vi "Red ball detection subVI.vi"(2 "error in":errorcluster, 3 "Image In":T1) -> (0 "error out":errorcluster, 1 "Image overlay":T1(plugin-control))   [LabVIEW 2018]
uses:
  <vilib>/vision/Image Controls.llb/IMAQ Image.ctl
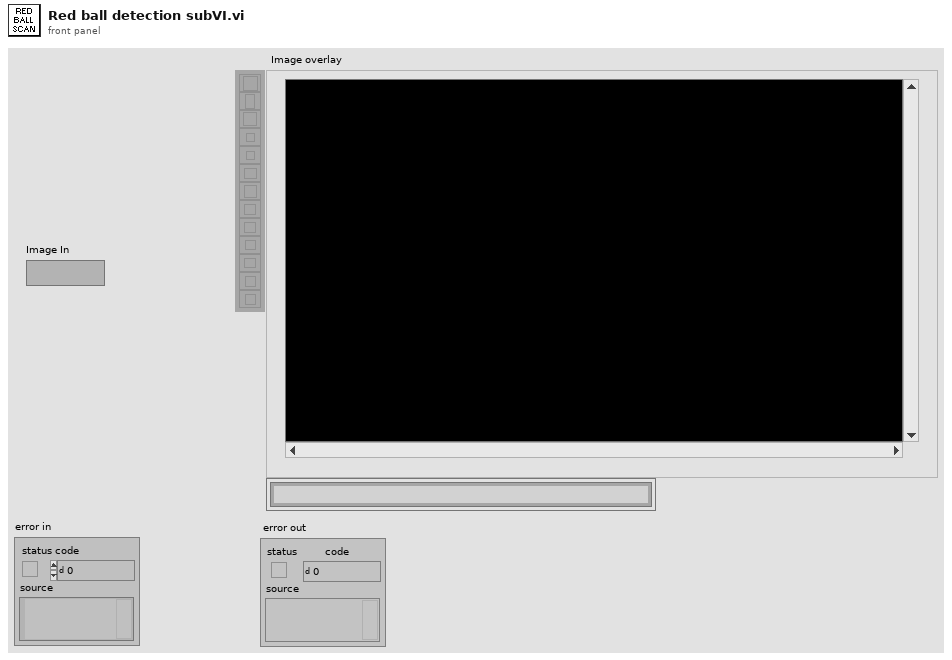
[diagram p1: front panel]
types:
  T1 = typedef "IMAQ Image.ctl" = refnum<image>
  T2 = cluster{"Desired Font (Application)":enum16{"User-specified Font", "Application Font", "System Font", "Dialog Font"}, "[User-specified Font]":cluster{"Font Name":string, "Size":i16, "Strikeout?":bool, "Italic?":bool, "Underline?":bool, "Outline?":bool, "Shadow?":bool, "Bold?":bool, "Rotation Angle":dbl}, "Horizontal Alignment":i16, "Vertical Alignment":i16}
  T3 = cluster{"Position":cluster{"x":sgl, "y":sgl}, "Angle":sgl, "Scale":sgl, "Score":sgl, "Bounding Box":cluster{"x":sgl, "y":sgl}[]}[]
  T4 = cluster{"Matches (Detect red)[0]":cluster{"Position":cluster{"x":sgl, "y":sgl}, "Angle":sgl, "Scale":sgl, "Score":sgl, "Bounding Box":cluster{"x":sgl, "y":sgl}[]}, "Matches (Detect red)[1]":cluster{"Position":cluster{"x":sgl, "y":sgl}, "Angle":sgl, "Scale":sgl, "Score":sgl, "Bounding Box":cluster{"x":sgl, "y":sgl}[]}, "Matches (Detect red)[2]":cluster{"Position":cluster{"x":sgl, "y":sgl}, "Angle":sgl, "Scale":sgl, "Score":sgl, "Bounding Box":cluster{"x":sgl, "y":sgl}[]}, "Matches (Detect red)[3]":cluster{"Position":cluster{"x":sgl, "y":sgl}, "Angle":sgl, "Scale":sgl, "Score":sgl, "Bounding Box":cluster{"x":sgl, "y":sgl}[]}, "Matches (Detect red)[4]":cluster{"Position":cluster{"x":sgl, "y":sgl}, "Angle":sgl, "Scale":sgl, "Score":sgl, "Bounding Box":cluster{"x":sgl, "y":sgl}[]}, "Matches (Detect red)[5]":cluster{"Position":cluster{"x":sgl, "y":sgl}, "Angle":sgl, "Scale":sgl, "Score":sgl, "Bounding Box":cluster{"x":sgl, "y":sgl}[]}, "Matches (Detect red)[6]":cluster{"Position":cluster{"x":sgl, "y":sgl}, "Angle":sgl, "Scale":sgl, "Score":sgl, "Bounding Box":cluster{"x":sgl, "y":sgl}[]}, "Matches (Detect red)[7]":cluster{"Position":cluster{"x":sgl, "y":sgl}, "Angle":sgl, "Scale":sgl, "Score":sgl, "Bounding Box":cluster{"x":sgl, "y":sgl}[]}, "Matches (Detect red)[8]":cluster{"Position":cluster{"x":sgl, "y":sgl}, "Angle":sgl, "Scale":sgl, "Score":sgl, "Bounding Box":cluster{"x":sgl, "y":sgl}[]}}
  T5 = cluster{"Bounding Box[0]":cluster{"x":sgl, "y":sgl}, "Bounding Box[1]":cluster{"x":sgl, "y":sgl}, "Bounding Box[2]":cluster{"x":sgl, "y":sgl}, "Bounding Box[3]":cluster{"x":sgl, "y":sgl}, "Bounding Box[4]":cluster{"x":sgl, "y":sgl}, "Bounding Box[5]":cluster{"x":sgl, "y":sgl}, "Bounding Box[6]":cluster{"x":sgl, "y":sgl}, "Bounding Box[7]":cluster{"x":sgl, "y":sgl}, "Bounding Box[8]":cluster{"x":sgl, "y":sgl}}
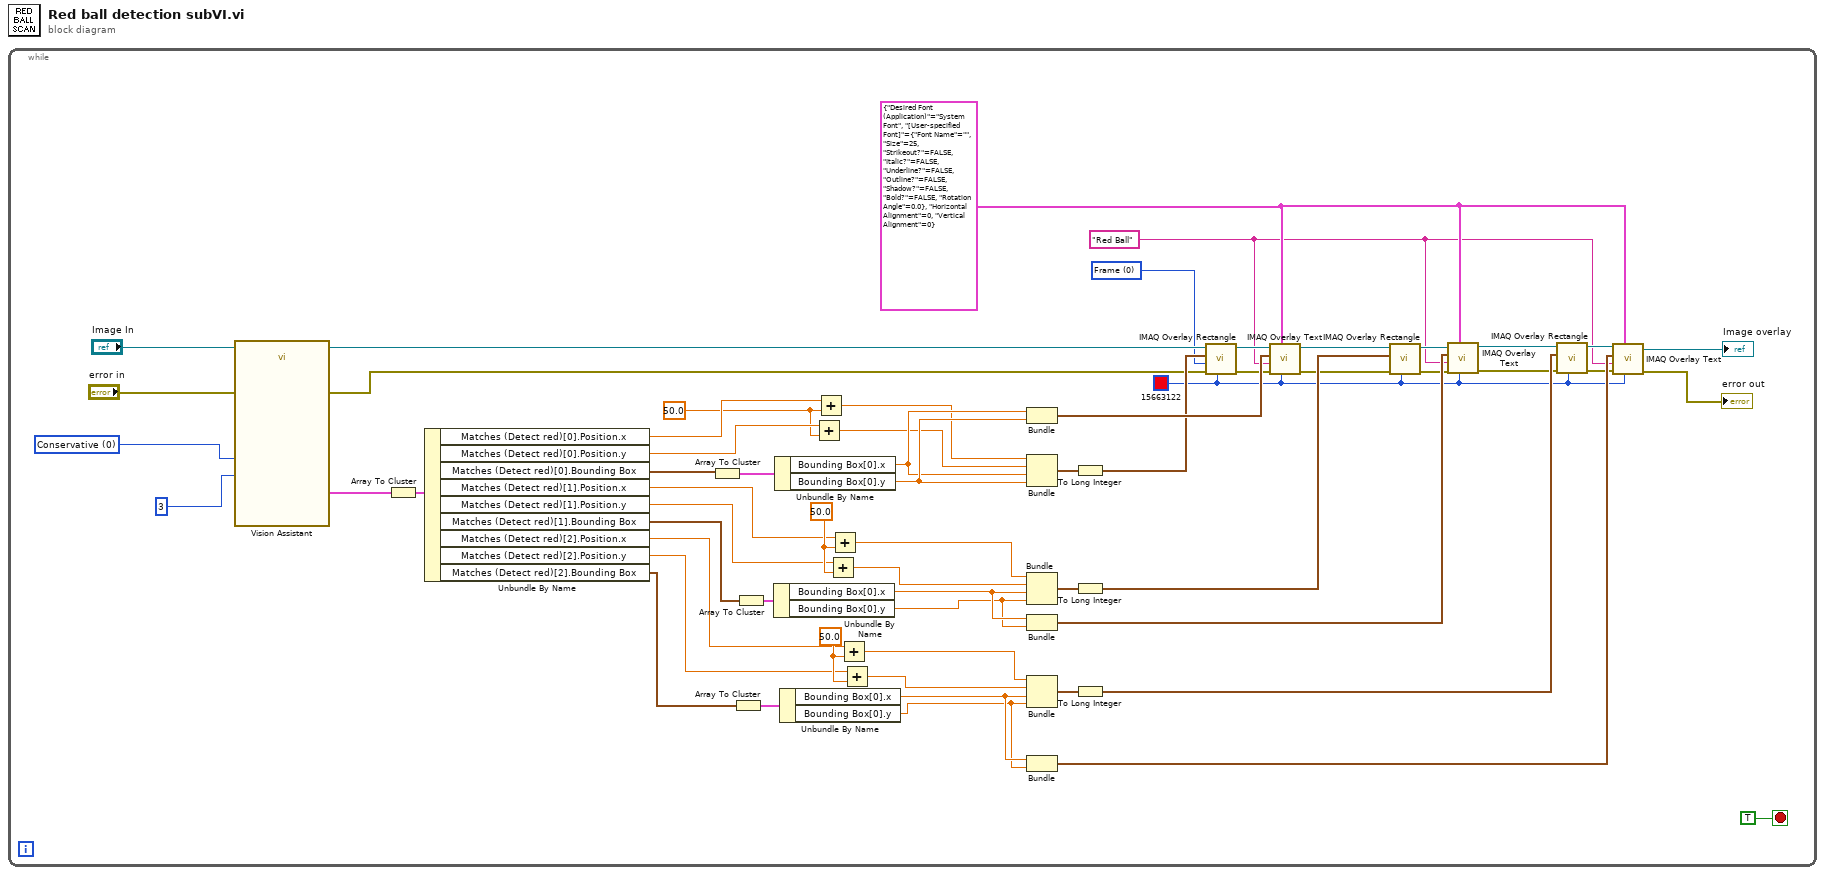
[diagram p0: block diagram]
diagram:
  n1 = while {
    stop <- TRUE stop-if-true
    w45 = u32 0 items=["Conservative", "Balance", "Aggressive", "Very Aggressive"] ("Search Strategy (Detect red)")
    w25 = sgl 50.0 ("y")
    w40 = sgl 50.0 ("y")
    w41 = sgl 50.0 ("y")
    w1 = u32 15663122 ("Text Color (black)")
    w13 = T2 {"Desired Font (Application)"=enum."System Font", "[User-specified Font]"={"Font Name"="", "Size"=25, "Strikeout?"=FALSE, "Italic?"=FALSE, "Underline?"=FALSE, "Outline?"=FALSE, "Shadow?"=FALSE, "Bold?"=FALSE, "Rotation Angle"=0.0}, "Horizontal Alignment"=0, "Vertical Alignment"=0} ("Font, Size & Style")
    w12 = "Red Ball" ("String")
    w33 = u32 0 items=["Frame", "Fill", "Highlight"] ("Drawing Mode (Frame)")
    n2 = call "Vision Assistant"("Image In"="Image In", "Search Strategy (Detect red)"=w45, "Number of Matches Requested (Detect red)"=3, "error in"="error in") -> ("Image Out"=w58:T1, "Matches (Detect red)"=w60:T3, "error out"=w2:errorcluster)  [unwired: 20 in, 1 out]
    n3 = Array To Cluster(array=w60) -> (cluster=w59:T4)
    n4 = Unbundle By Name(w59) -> ("Matches (Detect red)[0].Position.x"=w49:sgl, "Matches (Detect red)[0].Position.y"=w47:sgl, "Matches (Detect red)[0].Bounding Box"=w57:cluster{"x":sgl, "y":sgl}[], "Matches (Detect red)[1].Position.x"=w39:sgl, "Matches (Detect red)[1].Position.y"=w38:sgl, "Matches (Detect red)[1].Bounding Box"=w43:cluster{"x":sgl, "y":sgl}[], "Matches (Detect red)[2].Position.x"=w24:sgl, "Matches (Detect red)[2].Position.y"=w23:sgl, "Matches (Detect red)[2].Bounding Box"=w26:cluster{"x":sgl, "y":sgl}[])
    n5 = Array To Cluster(array=w57) -> (cluster=w56:T5)
    n6 = Array To Cluster(array=w26) -> (cluster=w27:T5)
    n7 = Array To Cluster(array=w43) -> (cluster=w42:T5)
    n8 = Unbundle By Name(w42) -> ("Bounding Box[0].x"=w30:sgl, "Bounding Box[0].y"=w29:sgl)
    n9 = Unbundle By Name(w56) -> ("Bounding Box[0].x"=w50:sgl, "Bounding Box[0].y"=w53:sgl)
    n10 = Unbundle By Name(w27) -> ("Bounding Box[0].x"=w19:sgl, "Bounding Box[0].y"=w18:sgl)
    n11 = Add(x=w47, y=w41) -> (x+y=w46:sgl)
    n12 = Add(x=w49, y=w41) -> (x+y=w48:sgl)
    n13 = Add(x=w38, y=w40) -> (x+y=w36:sgl)
    n14 = Add(x=w39, y=w40) -> (x+y=w37:sgl)
    n15 = Add(x=w24, y=w25) -> (x+y=w22:sgl)
    n16 = Add(x=w23, y=w25) -> (x+y=w21:sgl)
    n17 = Bundle("x"=w50, "y"=w53) -> (w54:cluster{"x":sgl, "y":sgl})  [unwired: 1 in]
    n18 = Bundle(w48, w46, "x"=w50, "y"=w53) -> (w52:cluster{sgl, sgl, "x":sgl, "y":sgl})  [unwired: 1 in]
    n19 = Bundle(w37, w36, "x"=w30, "y"=w29) -> (w35:cluster{sgl, sgl, "x":sgl, "y":sgl})  [unwired: 1 in]
    n20 = Bundle("x"=w30, "y"=w29) -> (w28:cluster{"x":sgl, "y":sgl})  [unwired: 1 in]
    n21 = Bundle(w22, w21, "x"=w19, "y"=w18) -> (w20:cluster{sgl, sgl, "x":sgl, "y":sgl})  [unwired: 1 in]
    n22 = Bundle("x"=w19, "y"=w18) -> (w14:cluster{"x":sgl, "y":sgl})  [unwired: 1 in]
    n23 = To Long Integer(number=w52) -> (32bit integer=w51:cluster{i32, i32, "x":i32, "y":i32})
    n24 = To Long Integer(number=w35) -> (32bit integer=w34:cluster{i32, i32, "x":i32, "y":i32})
    n25 = To Long Integer(number=w20) -> (32bit integer=w16:cluster{i32, i32, "x":i32, "y":i32})
    n26 = call "IMAQ Overlay Rectangle"("Color"=w1, "error in (no error)"=w2, "Drawing Mode (Frame)"=w33, "Rectangle"=w51, "Image"=w58) -> ("error out"=w11:errorcluster, "Image Out"=w55:T1)  [unwired: 5 in]
    n27 = call "IMAQ Overlay Text"("Text Color (black)"=w1, "Font, Size & Style"=w13, "error in (no error)"=w11, "String"=w12, "Origin"=w54, "Image"=w55) -> ("error out"=w10:errorcluster, "Image Out"=w31:T1)  [unwired: 4 in]
    n28 = call "IMAQ Overlay Rectangle"("Color"=w1, "error in (no error)"=w10, "Rectangle"=w34, "Image"=w31) -> ("error out"=w9:errorcluster, "Image Out"=w32:T1)  [unwired: 6 in]
    n29 = call "IMAQ Overlay Text"("Text Color (black)"=w1, "Font, Size & Style"=w13, "error in (no error)"=w9, "String"=w12, "Origin"=w28, "Image"=w32) -> ("error out"=w8:errorcluster, "Image Out"=w17:T1)  [unwired: 4 in]
    n30 = call "IMAQ Overlay Rectangle"("Color"=w1, "error in (no error)"=w8, "Rectangle"=w16, "Image"=w17) -> ("error out"=w7:errorcluster, "Image Out"=w15:T1)  [unwired: 6 in]
    n31 = call "IMAQ Overlay Text"("Text Color (black)"=w1, "Font, Size & Style"=w13, "error in (no error)"=w7, "String"=w12, "Origin"=w14, "Image"=w15) -> ("error out"=→"error out":errorcluster, "Image Out"=→"Image overlay":T1)  [unwired: 4 in]
  }
